vi "RequestRegTemplate.vi"(8 "error in (no error)":errorcluster) -> (0 "error out":errorcluster, 3 "user event out":refnum<user-event>)   [LabVIEW 2024, in "AddNewEvent.lvlib"]
uses:
  AddNewEvent.lvlib
  RQMHCore/ModuleCore/Reply.ctl
  RQMHCore/ModuleCore/Module.lvclass
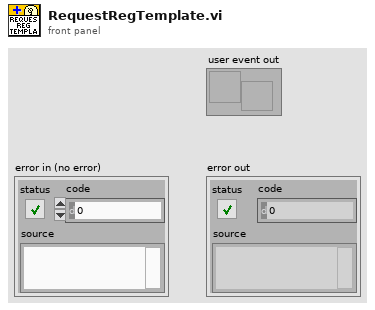
[diagram p1: front panel]
types:
  T1 = typedef "Module.lvclass/Reply.ctl" = cluster{"Expects Reply":bool, "Reply":refnum<notifier>}
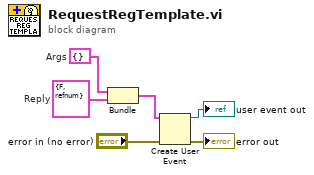
[diagram p0: block diagram]
diagram:
  w4 = cluster{} {}  # Args
  w3 = T1 {"Expects Reply"=FALSE, "Reply"=refnum}  # Reply
  n1 = Bundle("Args"=w4, "Reply"=w3) -> (w2:cluster{"Args":cluster{}, "Reply":T1})  [unwired: 1 in]
  n2 = Create User Event(user event datatype=w2, error in="error in (no error)") -> (user event=→"user event out":refnum<user-event>, error out=→"error out":errorcluster)
